vi "arduino_servo_intensidad.vi"() -> ()   [LabVIEW 2017]
uses:
  <vilib>/Instr/_visa.llb/VISA Configure Serial Port (Instr).vi
  <vilib>/Utility/file.llb/Write Delimited Spreadsheet (DBL).vi
panel:
  out "Máxima intensidad registrada 2":dbl
  out "Angulo intensidad máxima 2":dbl
  in  "Valsor máximo":bool
  in  "Muestreo de intensidad":bool
  out "Angulo intensidad máxima":dbl
  out "Indice":i32
  out "Máxima intensidad registrada":dbl
  in  "file path (use dialog)":path=path "C:/"
  out "XY Graph":cluster{"Y":dbl[], "Y":dbl[]}[](graph)
  in  "stop":bool
  out "Angulo":dbl
  out "Intensidad":dbl
  in  "INICIO":bool
  in  "VISA resource name":refnum<visa-resource-name>
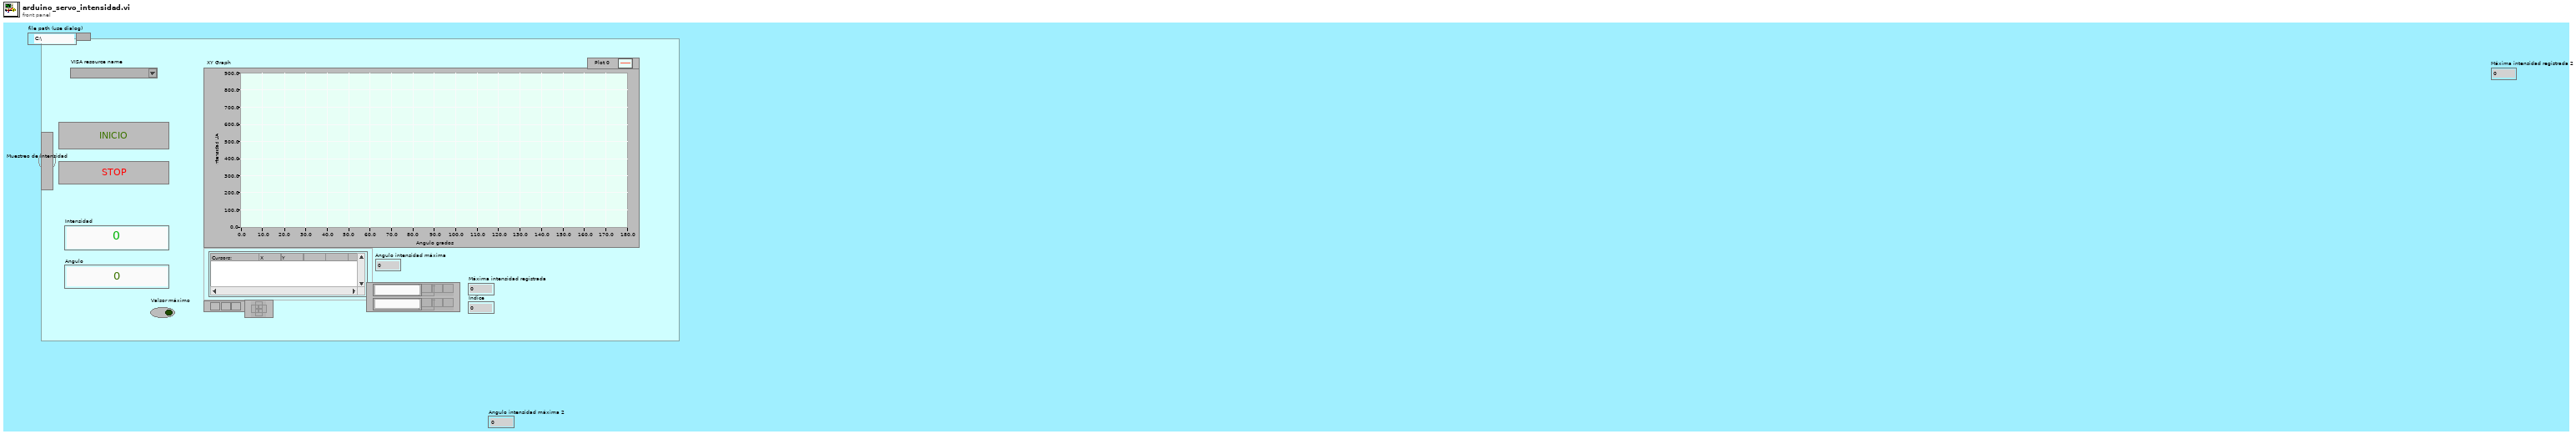
[diagram p1: front panel]
types:
  T1 = enum16{"open", "replace", "create", "open or create", "replace or create", "replace or create with confirmation"}
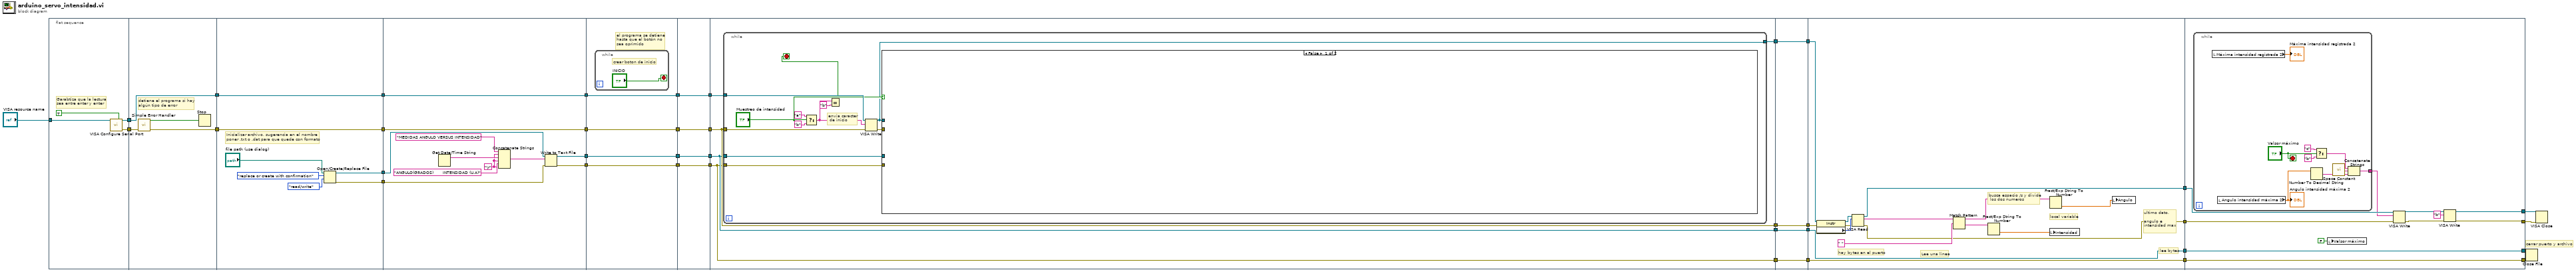
[diagram p0: block diagram]
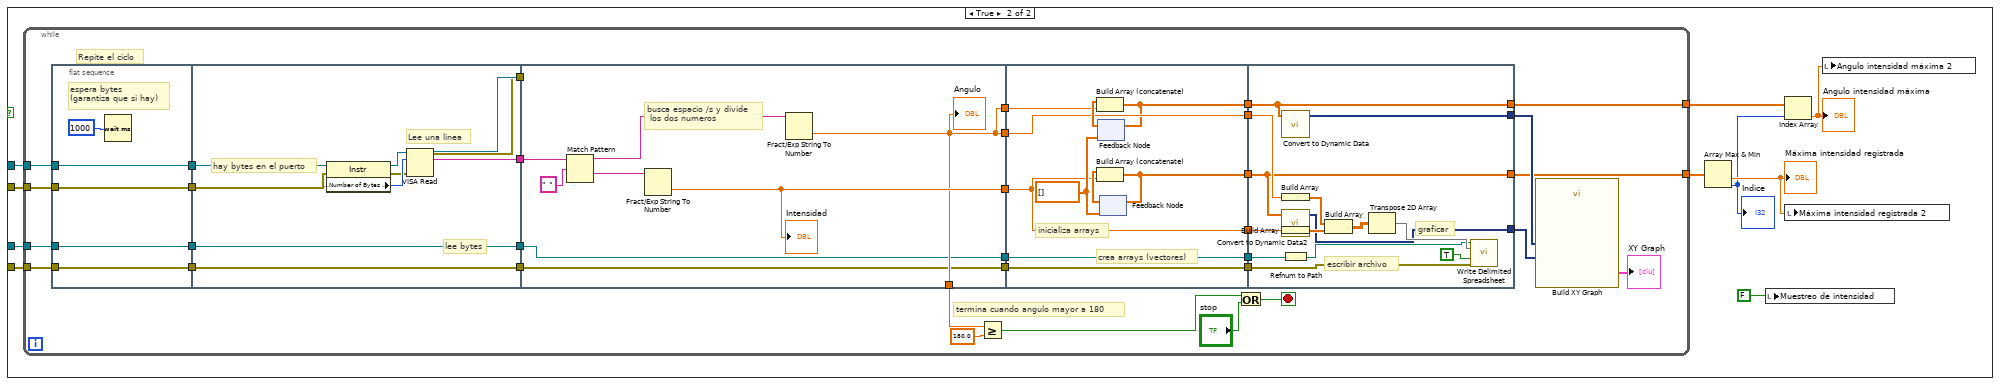
[diagram p2: hidden frame]
diagram:
  # "cerrar puerto y archivo"
  n1 = flat-sequence {
    tunnel: "VISA resource name" -> [w41]
    tunnel: [w39] -> w36
    tunnel: [w38] -> w35
    tunnel: w36 -> [w42]
    tunnel: w35 -> [w45]
    tunnel: [w42] -> w34
    tunnel: [w43] -> w33
    tunnel: w34 -> [w52]
    tunnel: w33 -> [w51]
    tunnel: [w52] -> w32
    tunnel: [w51] -> w30
    tunnel: [w47] -> w28
    tunnel: [w46] -> w27
    tunnel: w32 -> [w63]
    tunnel: [w63] -> w31
    tunnel: w30 -> [w62]
    tunnel: [w62] -> w29
    tunnel: w28 -> [w55]
    tunnel: w27 -> [w57]
    tunnel: [w54] -> w26
    tunnel: [w53] -> w25
    tunnel: w31 -> [w67]
    tunnel: w29 -> [w66]
    tunnel: w26 -> [w65]
    tunnel: w25 -> [w64]
    tunnel: [w67] -> w24
    tunnel: [w66] -> w22
    tunnel: [w65] -> w20
    tunnel: [w64] -> w18
    tunnel: w24 -> [w70]
    tunnel: [w70] -> w23
    tunnel: w22 -> [w69]
    tunnel: [w69] -> w21
    tunnel: w20 -> [w72]
    tunnel: [w72] -> w19
    tunnel: w18 -> [w71]
    tunnel: [w71] -> w17
    tunnel: w23 -> [w74]
    tunnel: w21 -> [w77]
    tunnel: w19 -> [w76]
    tunnel: w17 -> [w75]
    tunnel: [w73] -> w10
    tunnel: [w77] -> w8
    tunnel: [w76] -> w6
    tunnel: [w75] -> w4
    tunnel: w10 -> [w184]
    tunnel: [w184] -> w9
    tunnel: w8 -> [w183]
    tunnel: [w183] -> w7
    tunnel: w6 -> [w182]
    tunnel: [w182] -> w5
    tunnel: w4 -> [w181]
    tunnel: [w181] -> w3
    tunnel: w9 -> [w191]
    tunnel: w7 -> [w190]
    tunnel: w5 -> [w199]
    tunnel: w3 -> [w198]
    tunnel: [w199] -> w16
    tunnel: [w198] -> w15
    tunnel: [w189] -> w14
    tunnel: [w188] -> w13
    tunnel: w16 -> [w209]
    tunnel: w15 -> [w210]
    tunnel: w14 -> [w208]
    tunnel: w13 -> [w206]
    tunnel: [w210] -> w12
    tunnel: [w209] -> w11
    tunnel: [w201] -> w2
    tunnel: [w202] -> w1
    frame #0 {
      # "Garabtiza que la lectura \nsea entre enter y enter"
      n2 = call-poly "VISA Configure Serial Port"("VISA resource name"=w41, "Enable Termination\nChar (T)"=TRUE ("Enable Termination\nChar (T)")) -> ("VISA resource name out"=w39:refnum<visa-resource-name>, "error out"=w38:errorcluster)  [unwired: 12 in]
    }
    frame #1 {
      # "detiene el programa si hay \nalgún tipo de error"
      n3 = call <vilib>:"Simple Error Handler.vi"("error in (no error)"=w45) -> ("error?"=w44:bool, "error out"=w43:errorcluster)  [unwired: 4 in, 3 out]
      n4 = Stop(stop? (T)=w44) -> ()
    }
    frame #2 {
      # "Inicializar archivo, sugerencia en el nombre\nponer .txt o .dat para que quede con formato"
      n5 = Open/Create/Replace File(file path (use dialog)="file path (use dialog)", operation (0:open)=T1."replace or create with confirmation", access (0:read/write)=enum16{"read/write", "read-only", "write-only"}."read/write") -> (refnum out=w46:refnum<file>, error out=w47:errorcluster)  [unwired: 3 in, 1 out]
    }
    frame #3 {
      w58 = "\r"
      n6 = Get Date/Time String() -> (date string=w60:string)  [unwired: 3 in, 1 out]
      n7 = Concatenate Strings "Concatenate Strings"("MEDIDAS ANGULO VERSUS INTENSIDAD", w58, w60, w58, "ANGULO(GRADOS)       INTENSIDAD (U.A)", w58) -> (w56:string)
      n8 = Write to Text File(file (use dialog)=w57, text=w56, error in=w55) -> (refnum out=w54:refnum<file>, error out=w53:errorcluster)  [unwired: 1 in, 1 out]
    }
    frame #4 {
      # "el programa se detiene \nhasta que el botón no \nsea oprimido"
      n9 = while {
        stop <- "INICIO" stop-if-true
        # "crear boton de inicio"
      }
    }
    frame #5 {
    }
    frame #6 {
      n10 = while {
        tunnel: w77 -> [w85]
        tunnel: w76 -> [w89]
        tunnel: w75 -> [w88]
        tunnel: w74 -> [w87]
        tunnel: [w81] -> w73
        stop <- w78 stop-if-true
        # "envia caracter\n de inicio"
        n11 = Select(t="a", s="Muestreo de intensidad", f="b") -> (s? t:f=w79:string)
        n12 = Equal?(x=w79, y="b") -> (x = y?=w78:bool)
        n13 = VISA Write(VISA resource name=w87, write buffer=w79, error in (no error)=w85) -> (VISA resource name out=w81:refnum<visa-resource-name>, error out=w86:errorcluster)  [unwired: 1 out]
        n14 = case shown="False" "Muestreo de intensidad" {
          tunnel: w89 -> [_ w99]
          tunnel: w88 -> [_ w98]
          tunnel: w86 -> [_ w97]
          tunnel: w81 -> [_ w96]
          frame False {
          }
          frame True {
            n15 = while {
              tunnel: w97 -> [w133]
              tunnel: w99 -> [w113]
              tunnel: w98 -> [w108]
              tunnel: w96 -> [w102]
              tunnel: [w101] -> w92
              tunnel: [w100] -> w91
              stop <- w125 stop-if-true
              # "termina cuando angulo mayor a 180"
              # "Repite el ciclo"
              n16 = flat-sequence {
                tunnel: w133 -> [w137]
                tunnel: w102 -> [w138]
                tunnel: [w138] -> w132
                tunnel: [w137] -> w131
                tunnel: [w135] -> w114
                tunnel: w113 -> [w135]
                tunnel: [w134] -> w109
                tunnel: w108 -> [w134]
                tunnel: w132 -> [w148]
                tunnel: w131 -> [w147]
                tunnel: [w143] -> w130
                tunnel: [w142] -> w122
                tunnel: [w141] -> w121
                tunnel: [w140] -> w115
                tunnel: w114 -> [w140]
                tunnel: [w139] -> w110
                tunnel: w109 -> [w139]
                tunnel: w130 -> [w154]
                tunnel: [w151] -> w129
                tunnel: [w151] -> w124
                tunnel: [w152] -> w123
                tunnel: w122 -> [_]
                tunnel: w121 -> [_]
                tunnel: [w151] -> w119
                tunnel: [w150] -> w116
                tunnel: w115 -> [w150]
                tunnel: [w149] -> w111
                tunnel: w110 -> [w149]
                tunnel: w124 -> [w165]
                tunnel: w123 -> [w161]
                tunnel: [w162] -> w120
                tunnel: w119 -> [w162]
                tunnel: [w161] -> w118
                tunnel: [w160] -> w117
                tunnel: w116 -> [w160]
                tunnel: [w159] -> w112
                tunnel: w111 -> [w159]
                tunnel: [w158] -> w107
                tunnel: [w157] -> w106
                tunnel: w120 -> [w180]
                tunnel: w118 -> [w179]
                tunnel: w117 -> [w173]
                tunnel: w112 -> [w172]
                tunnel: w107 -> [w168]
                tunnel: w106 -> [w167]
                tunnel: [w170] -> w105
                tunnel: [w169] -> w104
                tunnel: [w168] -> w101
                tunnel: [w167] -> w100
                frame #0 {
                  # "espera bytes \n(garantiza que si hay)"
                  n17 = Wait (ms)(milliseconds to wait=u32 1000) -> ()  [unwired: 1 out]
                }
                frame #1 {
                  # "lee bytes"
                  # "Lee una linea"
                  # "hay bytes en el puerto"
                  n18 = property class="Instr"(reference=w148, error in=w147) -> (reference out=w146:refnum<visa-resource-name>, error out=w144:errorcluster, "Serial Settings:Number of Bytes at Serial Port"=w145:u32)
                  n19 = VISA Read(VISA resource name=w146, byte count=w145, error in (no error)=w144) -> (VISA resource name out=w142:refnum<visa-resource-name>, read buffer=w143:string, error out=w141:errorcluster)  [unwired: 1 out]
                }
                frame #2 {
                  # "busca espacio /s y divide\n los dos numeros"
                  n20 = Match Pattern(string=w154, regular expression=" ") -> (before substring=w153:string, after substring=w156:string)  [unwired: 1 in, 2 out]
                  n21 = Fract/Exp String To Number(string=w156) -> (number=w152:dbl)  [unwired: 3 in, 1 out]
                  "Intensidad" <- w152
                  n22 = Fract/Exp String To Number(string=w153) -> (number=w151:dbl)  [unwired: 3 in, 1 out]
                  "Angulo" <- w151
                }
                frame #3 {
                  w163 = dbl[] []
                  # "inicializa arrays"
                  # "crea arrays (vectores)"
                  n23 = feedback #1(w163) -> (w166:dbl[])
                  n24 = Build Array (concatenate) "Build Array"(w166, w165) -> (w158:dbl[])
                  n25 = feedback-in #1(w158) -> ()
                  n26 = feedback #2(w163) -> (w164:dbl[])
                  n27 = Build Array (concatenate) "Build Array"(w164, w161) -> (w157:dbl[])
                  n28 = feedback-in #2(w157) -> ()
                }
                frame #4 {
                  # "graficar"
                  # "escribir archivo"
                  n29 = call "Convert to Dynamic Data"("Array"=w168) -> ("Dynamic Data Type"=w169:dynamicdata)  [unwired: 3 in]
                  n30 = Build Array(w180) -> (w178:dbl[])
                  n31 = call "Convert to Dynamic Data2"("Array"=w167) -> ("Dynamic Data Type"=w170:dynamicdata)  [unwired: 3 in]
                  n32 = Build Array(w179) -> (w177:dbl[])
                  n33 = Refnum to Path(1:w173) -> (0:w174:path)
                  n34 = Build Array(w178, w177) -> (w176:dbl[][])
                  n35 = Transpose 2D Array(2D array=w176) -> (transposed array=w175:dbl[][])
                  n36 = call-poly <vilib>:"Write Delimited Spreadsheet.vi"("file path (dialog if empty)"=w174, "2D data"=w175, "append to file? (new file:F)"=TRUE, "error in (no error)"=w172) -> ()  [unwired: 10 in, 2 out]
                }
              }
              n37 = Greater Or Equal?(x=w129, y=180.0) -> (x >= y?=w127:bool)
              n38 = Or(x=w127, y="stop") -> (x .or. y?=w125:bool)
              n39 = call "Build XY Graph"("Y Input"=w105, "X Input"=w104) -> ("XY Graph"=→"XY Graph":cluster{"X":dbl[], "Y":dbl[]}[])  [unwired: 8 in, 1 out]
            }
            n40 = Array Max & Min(array=w91) -> (min value=w95:dbl, min index (indices)=w94:i32)  [unwired: 2 out]
            "Máxima intensidad registrada" <- w95
            "Indice" <- w94
            n41 = local write "Muestreo de intensidad"(FALSE ("Inicio omunicación serial 2")) -> ()
            n42 = Index Array(array=w92, index=w94) -> (element=w93:dbl)
            "Angulo intensidad máxima" <- w93
            n43 = local write "Máxima intensidad registrada 2"(w95) -> ()
            n44 = local write "Angulo intensidad máxima 2"(w93) -> ()
          }
        }
      }
    }
    frame #7 {
    }
    frame #8 {
      # "local variable"
      # "lee bytes"
      # "Lee una linea"
      # "hay bytes en el puerto"
      # "busca espacio /s y divide\n los dos numeros"
      # "ultimo dato, \n\nangulo e \nintensidad max"
      n45 = property class="Instr"(reference=w191, error in=w190) -> (reference out=w197:refnum<visa-resource-name>, error out=w195:errorcluster, "Serial Settings:Number of Bytes at Serial Port"=w196:u32)
      n46 = VISA Read(VISA resource name=w197, byte count=w196, error in (no error)=w195) -> (VISA resource name out=w189:refnum<visa-resource-name>, read buffer=w187:string, error out=w188:errorcluster)  [unwired: 1 out]
      n47 = Match Pattern(string=w187, regular expression=" ") -> (before substring=w192:string, after substring=w194:string)  [unwired: 1 in, 2 out]
      n48 = Fract/Exp String To Number(string=w194) -> (number=w185:dbl)  [unwired: 3 in, 1 out]
      n49 = Fract/Exp String To Number(string=w192) -> (number=w186:dbl)  [unwired: 3 in, 1 out]
      n50 = local write "Intensidad"(w185) -> ()
      n51 = local write "Angulo"(w186) -> ()
    }
    frame #9 {
      n52 = while {
        tunnel: [w214] -> w207
        stop <- "Valsor máximo" stop-if-true
        n53 = local read "Máxima intensidad registrada 2"() -> (→"Máxima intensidad registrada 2":dbl)
        n54 = local read "Angulo intensidad máxima 2"() -> (w216:dbl)
        "Angulo intensidad máxima 2" <- w216
        n55 = Number To Decimal String(number=w216) -> (decimal integer string=w211:string)  [unwired: 1 in]
        n56 = Select(t="c", s="Valsor máximo", f="b") -> (s? t:f=w215:string)
        n57 = call <vilib>:"Space Constant.vi"() -> ("String"=w213:string)
        n58 = Concatenate Strings(w215, w213, w211) -> (w214:string)
      }
      n59 = local write "Valsor máximo"(FALSE ("Valsor máximo")) -> ()
      n60 = VISA Write(VISA resource name=w208, write buffer=w207, error in (no error)=w206) -> (VISA resource name out=w204:refnum<visa-resource-name>, error out=w203:errorcluster)  [unwired: 1 out]
      n61 = VISA Write(VISA resource name=w204, write buffer="b", error in (no error)=w203) -> (VISA resource name out=w202:refnum<visa-resource-name>, error out=w201:errorcluster)  [unwired: 1 out]
    }
  }
  n62 = Close File(refnum=w11, error in=w12) -> ()  [unwired: 2 out]
  n63 = VISA Close(VISA resource name=w1, error in (no error)=w2) -> ()  [unwired: 1 out]
